vi "ClampNumberTo0-25.vi"(1 "Number":dbl) -> (0 "Clamped number":dbl=25.0)   [LabVIEW 2013]
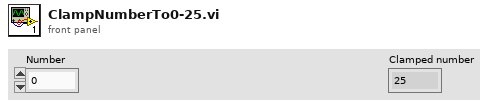
[diagram p1: front panel]
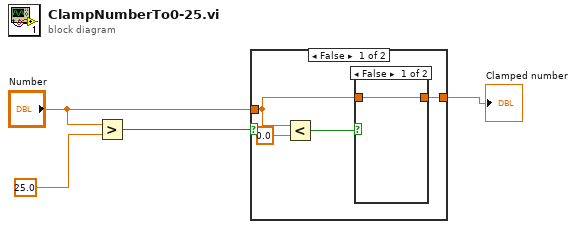
[diagram p0: block diagram]
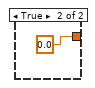
[diagram p2: hidden frame]
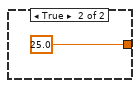
[diagram p3: hidden frame]
diagram:
  n1 = Greater?(x="Number", y=25.0) -> (0:w4:bool)
  n2 = case shown="False" w4 {
    tunnel: [w6 25.0] -> w2
    tunnel: "Number" -> [w5 _]
    frame False {
      n3 = Less?(x=w5, y=0.0) -> (x < y?=w7:bool)
      n4 = case shown="False" w7 {
        tunnel: [w9 0.0] -> w6
        tunnel: w5 -> [w9 _]
        frame False {
        }
        frame True {
        }
      }
    }
    frame True {
    }
  }
  "Clamped number" <- w2
